vi "_CSMObj-Obtain Chain.vi"(8 "Error in":errorcluster caption="Error in (no error)", 11 "Requested Name":string) -> (0 "Error out":errorcluster, 3 "CSMQ out":T1={"Requested Name"="", "Module Name"="", "Mode"=enum."Stand Alone", "Queue"=refnum, "CSM-Data"=refnum, "User Event"=refnum, "Status Change Event"=refnum, "Allowed Messages"=[], "Mode-Data"=refnum, "Group Name"="", "Exit Event"=refnum})   [LabVIEW 2020, in "Communicable State Machine.lvlib"]
uses:
  Communicable State Machine.lvlib
  _CSMObj.ctl
  Priority Queue.lvclass
  _CSM_MODE.ctl
  _CSMObj-Data.ctl
  _CSM Status Change Event Data.ctl
  _CSMObj-ModeData.ctl
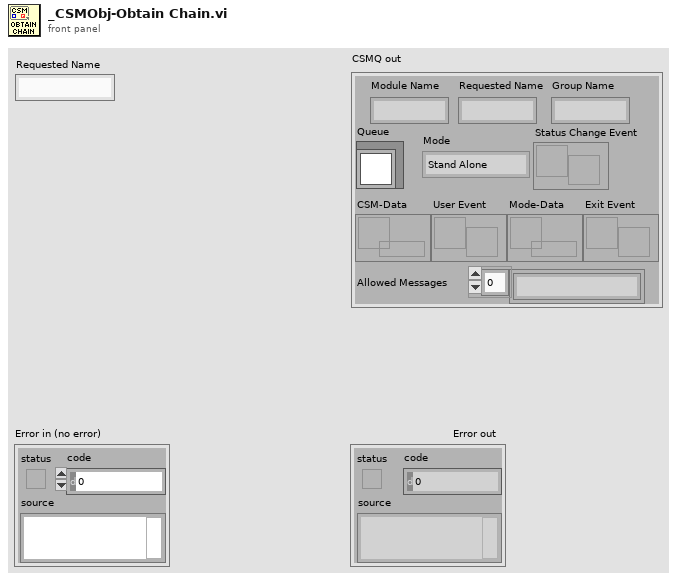
[diagram p1: front panel]
types:
  T1 = typedef "Communicable State Machine.lvlib/_CSMObj.ctl" = cluster{"Requested Name":string, "Module Name":string, "Mode":T2, "Queue":refnum<class "Priority Queue.lvclass">, "CSM-Data":refnum<data-value>, "User Event":refnum<user-event>, "Status Change Event":refnum<user-event>, "Allowed Messages":string[], "Mode-Data":refnum<data-value>, "Group Name":string, "Exit Event":refnum<user-event>}
  T2 = typedef "Communicable State Machine.lvlib/_CSM_MODE.ctl" = enum16{"Not Exist", "Stand Alone", "CSM", "Worker Agent", "Worker", "Chain", "Chain Node"}
  T3 = typedef "Communicable State Machine.lvlib/_CSMObj-ModeData.ctl" = cluster{"Share Count":i32, "Messages of Chain Nodes":cluster{"Module Name":string, "Allowed Messages":string[]}[], "Chain Message Mapping Map":variant}
  T4 = typedef "Communicable State Machine.lvlib/_CSMObj-Data.ctl" = cluster{"RemoteMessge?":bool, "error":errorcluster}
  T5 = typedef "Communicable State Machine.lvlib/_CSM Status Change Event Data.ctl" = cluster{"ModuleName":string, "Status":string, "Arguments":string}
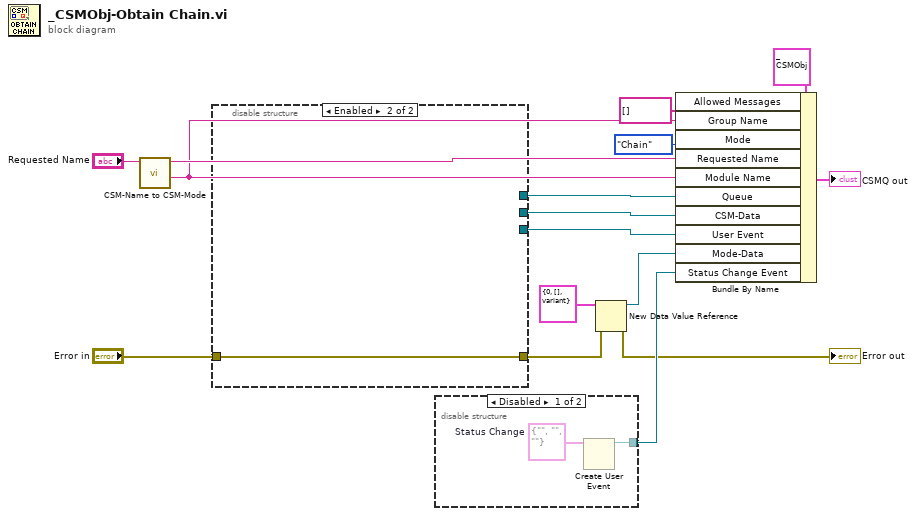
[diagram p0: block diagram]
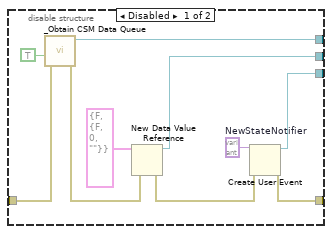
[diagram p2: hidden frame]
diagram:
  n1 = call "CSM-Name to CSM-Mode.vi"("String"="Requested Name") -> ("ParentCSM Name"=w4:string, "Requested Name"=w8:string)  [unwired: 8 in, 1 out]
  n2 = disable-structure shown="Enabled" {
    disable-tunnel: [w26 _] -> w16
    disable-tunnel: [w25 _] -> w15
    disable-tunnel: [w22 _] -> w14
    disable-tunnel: "Error in" -> [w21 w27]
    disable-tunnel: [w20 w27] -> w6
    frame Disabled {
      w24 = variant  # NewStateNotifier
      n3 = call "_Obtain CSM Data Queue.vi"("error in (no error)"=w21, "create if not found? (T)"=TRUE) -> ("error out"=w19:errorcluster, "Priority Queue"=w26:refnum<class "Priority Queue.lvclass">)  [unwired: 7 in, 1 out]
      n4 = New Data Value Reference(data value=T4 {"RemoteMessge?"=FALSE, "error"={"status"=FALSE, "code"=0, "source"=""}} ("CSMObj-Data"), error in=w19) -> (data value reference=w25:refnum<data-value>, error out=w23:errorcluster)
      n5 = Create User Event(user event datatype=w24, error in=w23) -> (user event=w22:refnum<user-event>, error out=w20:errorcluster)
    }
    frame Enabled {
    }
  }
  n6 = disable-structure shown="Disabled" {
    disable-tunnel: [w28 _] -> w13
    frame Disabled {
      w29 = T5 {"ModuleName"="", "Status"="", "Arguments"=""}  # Status Change
      n7 = Create User Event(user event datatype=w29) -> (user event=w28:refnum<user-event>)  [unwired: 1 in, 1 out]
    }
    frame Enabled {
    }
  }
  n8 = New Data Value Reference(data value=T3 {"Share Count"=0, "Messages of Chain Nodes"=[], "Chain Message Mapping Map"=variant} ("CSMObj-Data"), error in=w6) -> (data value reference=w7:refnum<data-value>, error out=→"Error out":errorcluster)
  n9 = Bundle By Name(cluster=T1 {"Requested Name"="", "Module Name"="", "Mode"=enum."Stand Alone", "Queue"=refnum, "CSM-Data"=refnum, "User Event"=refnum, "Status Change Event"=refnum, "Allowed Messages"=[], "Mode-Data"=refnum, "Group Name"="", "Exit Event"=refnum} ("CSMQ in"), "Allowed Messages"=string[] [], "Group Name"=w4, "Mode"=_CSM_MODE."Chain", "Requested Name"=w8, "Module Name"=w4, "Queue"=w16, "CSM-Data"=w15, "User Event"=w14, "Mode-Data"=w7, "Status Change Event"=w13) -> (→"CSMQ out":T1)
